vi "Draw Expanded Terminals.vi"(7 "State":T1={"Worker Library Path"=path "", "Block Label"="", "Types"=[], "Selections"=[], "Icon"={"image type"=0, "image depth"=0, "image"=[], "mask"=[], "colors"=[], "Rectangle"={"left"=0, "top"=0, "right"=0, "bottom"=0}}, "Errors"={"Terminals"=[], "Generate"={"status"=FALSE, "code"=0, "source"=""}, "General"={"status"=FALSE, "code"=0, "source"=""}}, "Calculated Sizes"={"Block Width"=0, "Block Height"=0, "Half Width"=0, "Icon Top"=0, "Icon Bottom"=0, "Label Width"=0, "Half Label"=0, "Label Top"=0, "Text Width"=0, "Half Text"=0, "Text Height"=0, "Label Height"=0, "Expanded Width"=0, "Label Bottom"=0, "Expanded Top"=0, "Expanded Bottom"=0, "Expanded Height"=0, "Min Height"=0, "Max Height"=0}, "Special Terminal Indices"={"Action"=-1, "Init"=-1, "Tag"=-1, "State in"=-1, "State out"=-1, "Error"=-1, "Control"=-1, "Config"=-1}, "Terminals"=[], "Temp VI Name"="", "Description"="", "Smol Mode"=FALSE}, 11 "Picture In":picture) -> (3 "Picture":picture)   [LabVIEW 2022 SP3, in "FlexBlocks Support.lvlib"]
uses:
  FlexBlocks Support.lvlib
  Flex Block/State.ctl
  Type Descriptor.ctl
  Terminal Direction.ctl
  Value Mode.ctl
  Special Terminal.ctl
  <vilib>/picture/picture.llb/imagedata.ctl
  XNode Errors.ctl
  Calculated Sizes.ctl
  Special Terminal Indices.ctl
  Terminal Status.ctl
  Terminal State.ctl
  Terminal Draw Style.ctl
  Flex Block/Flex Block.xnode
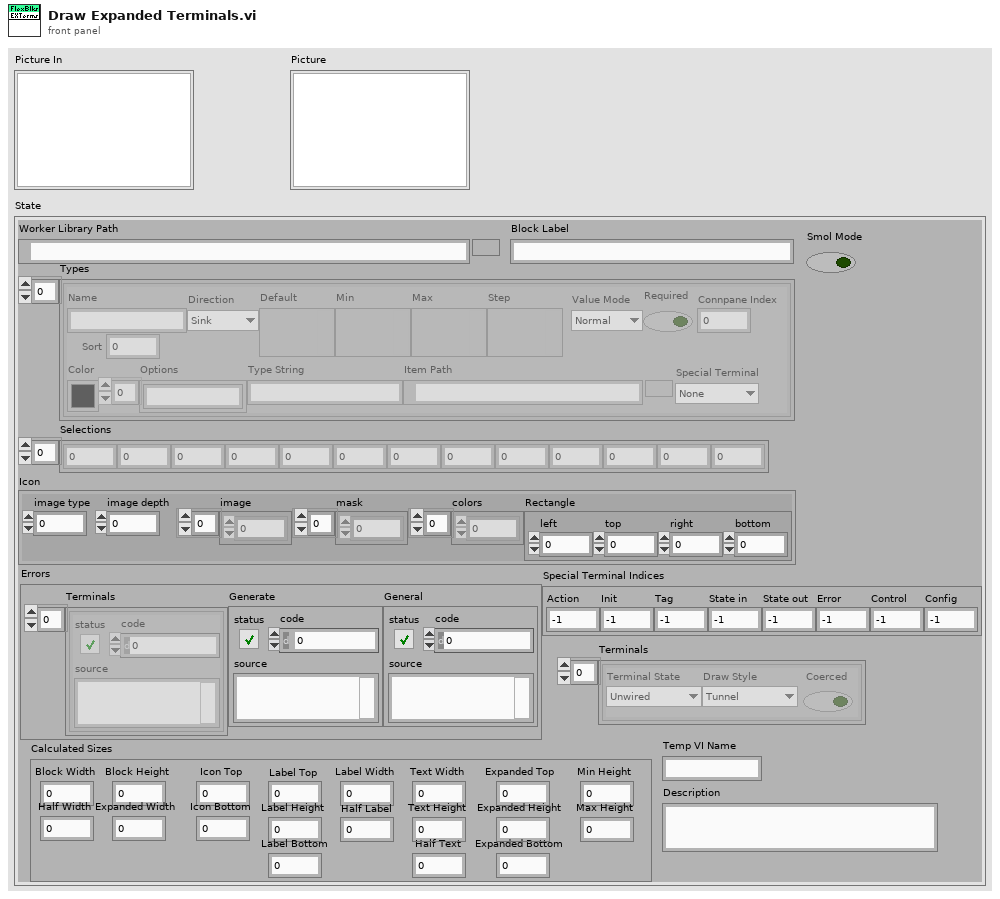
[diagram p1: front panel]
types:
  T1 = typedef "Flex Block.xnode/State.ctl" = cluster{"Worker Library Path":path, "Block Label":string, "Types":T2[], "Selections":i32[], "Icon":T6, "Errors":T7, "Calculated Sizes":T8, "Special Terminal Indices":T9, "Terminals":T10[], "Temp VI Name":string, "Description":string, "Smol Mode":bool}
  T2 = typedef "FlexBlocks Support.lvlib/Type Descriptor.ctl" = cluster{"Name":string, "Direction":T3, "Default":variant, "Min":variant, "Max":variant, "Step":variant, "Value Mode":T4, "Color":u32, "Options":string[], "Type String":string, "Item Path":path, "Required":bool, "Connpane Index":i32, "Special Terminal":T5, "Sort":i32}
  T3 = typedef "FlexBlocks Support.lvlib/Terminal Direction.ctl" = enum16{"Sink", "Source"}
  T4 = typedef "FlexBlocks Support.lvlib/Value Mode.ctl" = enum16{"Normal", "Range", "Select"}
  T5 = typedef "FlexBlocks Support.lvlib/Special Terminal.ctl" = enum16{"None", "Action", "Init", "Tag", "State in", "State out", "Error", "Control", "Config"}
  T6 = typedef "imagedata.ctl" = cluster{"image type":i32, "image depth":i32, "image":u8[], "mask":u8[], "colors":u32[], "Rectangle":cluster{"left":i16, "top":i16, "right":i16, "bottom":i16}}
  T7 = typedef "FlexBlocks Support.lvlib/XNode Errors.ctl" = cluster{"Terminals":errorcluster[], "Generate":errorcluster, "General":errorcluster}
  T8 = typedef "FlexBlocks Support.lvlib/Calculated Sizes.ctl" = cluster{"Block Width":i32, "Block Height":i32, "Half Width":i32, "Icon Top":i32, "Icon Bottom":i32, "Label Width":i32, "Half Label":i32, "Label Top":i32, "Text Width":i32, "Half Text":i32, "Text Height":i32, "Label Height":i32, "Expanded Width":i32, "Label Bottom":i32, "Expanded Top":i32, "Expanded Bottom":i32, "Expanded Height":i32, "Min Height":i32, "Max Height":i32}
  T9 = typedef "FlexBlocks Support.lvlib/Special Terminal Indices.ctl" = cluster{"Action":i32, "Init":i32, "Tag":i32, "State in":i32, "State out":i32, "Error":i32, "Control":i32, "Config":i32}
  T10 = typedef "FlexBlocks Support.lvlib/Terminal Status.ctl" = cluster{"Terminal State":T11, "Draw Style":T12, "Coerced":bool}
  T11 = typedef "FlexBlocks Support.lvlib/Terminal State.ctl" = enum16{"Unwired", "BadType", "BadRef", "Channel", "Value", "Control Ref"}
  T12 = typedef "FlexBlocks Support.lvlib/Terminal Draw Style.ctl" = enum16{"Tunnel", "BadType", "BadRef", "Channel", "Value", "Control Ref"}
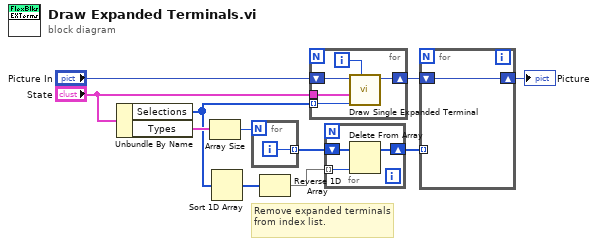
[diagram p0: block diagram]
diagram:
  # "Remove expanded terminals from index list."
  n1 = Unbundle By Name("State") -> ("Selections"=w1:i32[], "Types"=w5:T2[])
  n2 = Array Size(array=w5) -> (size(s)=w3:i32)
  n3 = Sort 1D Array(array=w1) -> (sorted array=w9:i32[])
  n4 = for {
    N: w3 -> [_]
    tunnel: [w12] -> w2 mode=indexing
    i -> [w12]
  }
  n5 = Reverse 1D Array(array=w9) -> (reversed array=w10:i32[])
  n6 = for {
    tunnel: w1 -> [w14] mode=indexing
    shift-right: [w16] -> w8
    shift-left: "Picture In" -> [w17]
    tunnel: "State" -> [w15]
    i -> [w13]
    n7 = call "Draw Single Expanded Terminal.vi"("Expanded Index"=w13, "Value Index"=w14, "State"=w15, "Picture In"=w17) -> ("Picture"=w16:picture)  [unwired: 7 in]
  }
  n8 = for {
    tunnel: w10 -> [w19] mode=indexing
    shift-right: [w18] -> w7
    shift-left: w2 -> [w20]
    n9 = Delete From Array(array=w20, index=w19) -> (array with subset deleted=w18:i32[])  [unwired: 1 in, 1 out]
  }
  n10 = for {
    tunnel: w7 -> [_] mode=indexing
    shift-right: [w21] -> w6
    shift-left: w8 -> [w21]
  }
  "Picture" <- w6
